vi "Measurement Logic.vi"() -> ()   [LabVIEW 2021, in "audio_acMeasurement.lvlib"]
uses:
  audio_acMeasurement.lvlib
  Measurement Configuration.ctl
  <vilib>/MeasurementLink/MeasurementLink Measurement Server/Classes/MeasurementContext/MeasurementContext.lvclass
  Measurement Results.ctl
  <vilib>/PDM Acquisition Toolkit/host/Classes/Tasks/PCM Input/Controls/DVR PCM Input Task.ctl
  <vilib>/PDM Acquisition Toolkit/host/Classes/Tasks/PCM Input/PCM Input Task.lvclass
  <vilib>/DAQmx/create/channels.llb/DAQmx Create Channel (AO-Voltage-Basic).vi
  <vilib>/DAQmx/configure/timing.llb/DAQmx Timing (Sample Clock).vi
  <vilib>/DAQmx/create/channels.llb/DAQmx Create Channel (AO-FuncGen).vi
  <vilib>/PDM Acquisition Toolkit/host/API/Public/Start/Start PCM Input Task.vi
  <vilib>/PDM Acquisition Toolkit/host/API/Public/Read/Read PCM Input Waveform.vi
  <vilib>/PDM Acquisition Toolkit/host/API/Public/Clear/Clear PCM Input Task.vi
  <resource>/objmgr/daqmx.rc
  <vilib>/PDM Acquisition Toolkit/host/API/PDM Acquisition Toolkit.lvlib
panel:
  out "Measurement Results":T1
  out "Measurement Context out":refnum<class "MeasurementContext.lvclass">
  in  "Measurement Context":refnum<class "MeasurementContext.lvclass">
  in  "Measurement Configuration":T2={"Band start"=20.0, "Band stop"=20000.0, "Weighting filter"=0, "Full scale range"=3.16, "Analog source resource name"="", "Frequency"=1000.0, "Amplitude"=1.0, "Protocol capture resource name"="PXI1Slot7\\I2Si 0", "Protocol capture channel"="", "Clock rate"=12288000, "Number of words"=19200, "Sensitivity"=0.34762, "JSONFile"=""}
  out "error out":errorcluster
  in  "error in":errorcluster
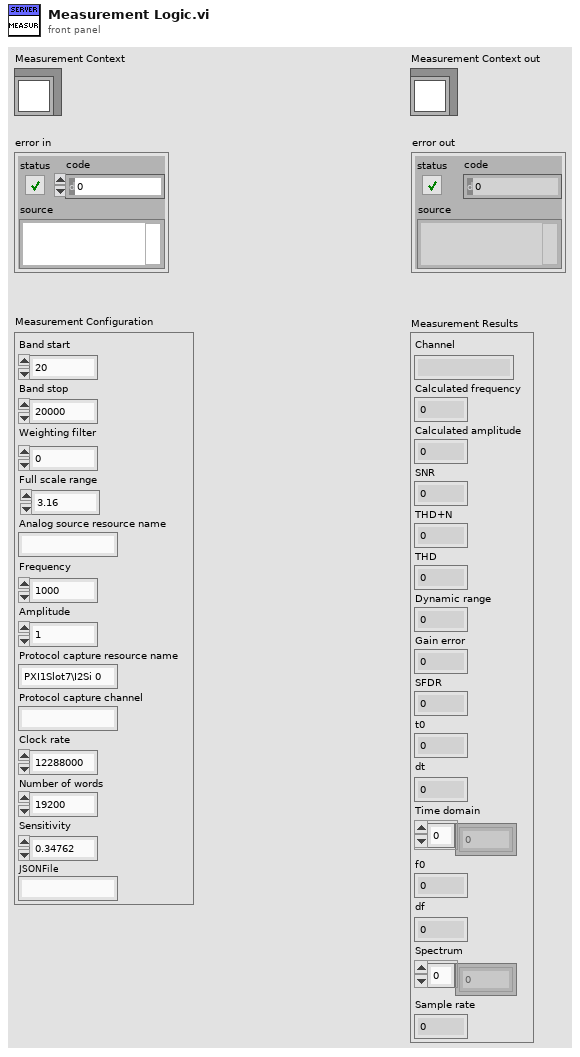
[diagram p1: front panel]
types:
  T1 = typedef "audio_acMeasurement.lvlib/Measurement Results.ctl" = cluster{"Channel":string, "Calculated frequency":dbl, "Calculated amplitude":dbl, "SNR":dbl, "THD+N":dbl, "THD":dbl, "Dynamic range":dbl, "Gain error":dbl, "SFDR":dbl, "t0":dbl, "dt":dbl, "Time domain":dbl[], "f0":dbl, "df":dbl, "Spectrum":dbl[], "Sample rate":u32}
  T2 = typedef "audio_acMeasurement.lvlib/Measurement Configuration.ctl" = cluster{"Band start":dbl, "Band stop":dbl, "Weighting filter":u16, "Full scale range":dbl, "Analog source resource name":string, "Frequency":dbl, "Amplitude":dbl, "Protocol capture resource name":string, "Protocol capture channel":string, "Clock rate":u32, "Number of words":u32, "Sensitivity":dbl, "JSONFile":string}
  T3 = typedef "PDM Acquisition Class Library.lvlib/PCM Input Task.lvclass/DVR PCM Input Task.ctl" = refnum<data-value>
  T4 = cluster{"DSG Session":refnum<k21>, "Calculated sample rate":u32, "PCM input task out":T3}
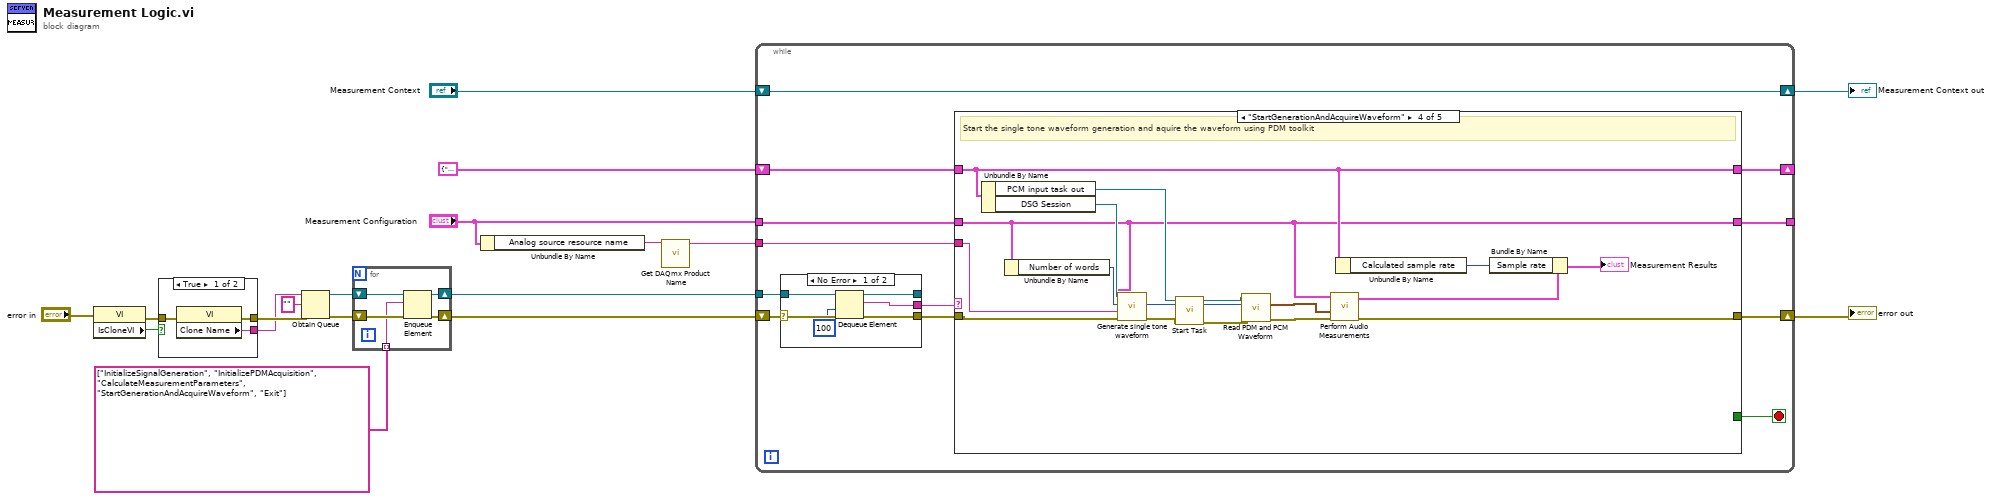
[diagram p0: block diagram]
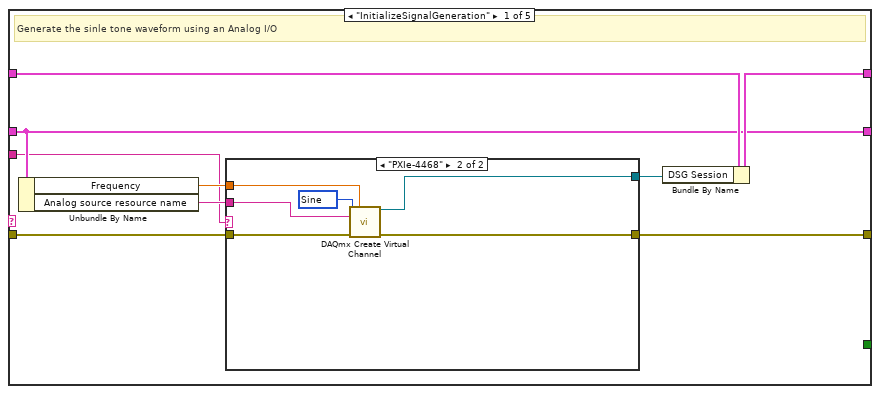
[diagram p2: hidden frame]
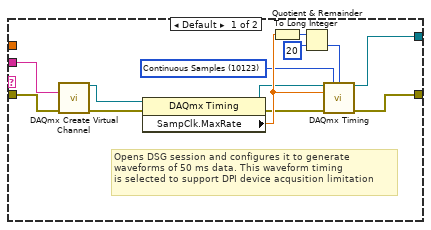
[diagram p3: hidden frame]
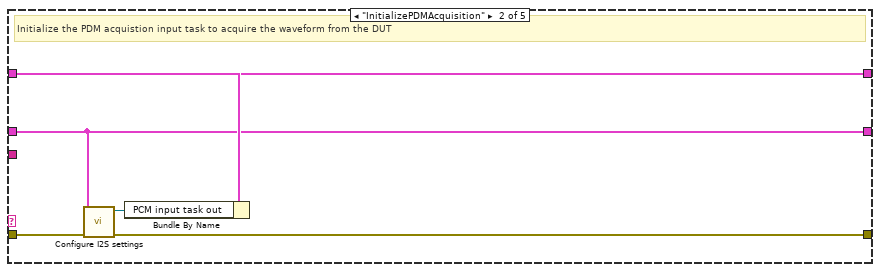
[diagram p4: hidden frame]
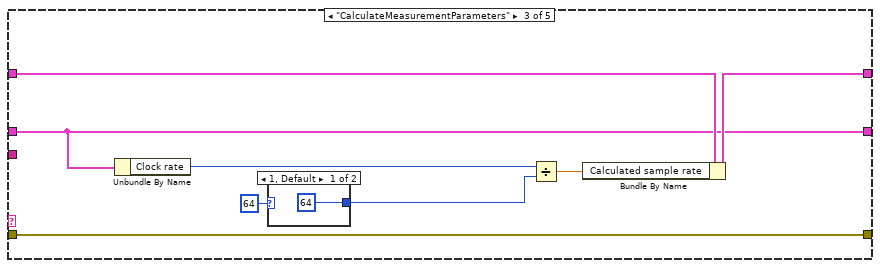
[diagram p5: hidden frame]
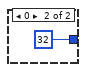
[diagram p6: hidden frame]
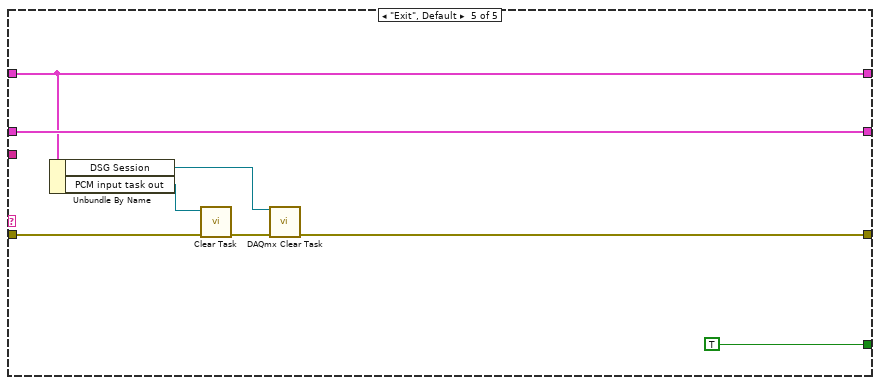
[diagram p7: hidden frame]
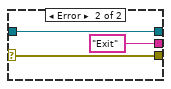
[diagram p8: hidden frame]
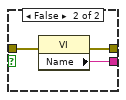
[diagram p9: hidden frame]
diagram:
  n1 = property class="VI"(error in="error in") -> (error out=w14:errorcluster, "IsCloneVI"=w15:bool)  [unwired: 1 in, 1 out]
  n2 = case shown="True" w15 {
    tunnel: [w21 w24] -> w13
    tunnel: [w20 w23] -> w12
    tunnel: w14 -> [w19 w22]
    frame True {
      n3 = property class="VI"(error in=w19) -> (error out=w21:errorcluster, "Clone Name"=w20:string)  [unwired: 1 in, 1 out]
    }
    frame False {
      n4 = property class="VI"(error in=w22) -> (error out=w24:errorcluster, "Name"=w23:string)  [unwired: 1 in, 1 out]
    }
  }
  n5 = Obtain Queue(name (unnamed)=w12, element data type="", error in (no error)=w13) -> (queue out=w17:refnum<queue>, error out=w11:errorcluster)  [unwired: 2 in, 1 out]
  n6 = for {
    shift-right: [w27] -> w10
    shift-left: w17 -> [w29]
    shift-right: [w26] -> w9
    shift-left: w11 -> [w28]
    tunnel: string[] ["InitializeSignalGeneration", "InitializePDMAcquisition", "CalculateMeasurementParameters", "StartGenerationAndAcquireWaveform", "Exit"] ("Step sequence") -> [w25] mode=indexing
    n7 = Enqueue Element(queue=w29, element=w25, error in (no error)=w28) -> (queue out=w27:refnum<queue>, error out=w26:errorcluster)  [unwired: 1 in, 1 out]
  }
  n8 = Unbundle By Name("Measurement Configuration") -> ("Analog source resource name"=w3:string)
  n9 = call "Get DAQmx Product Name.vi"("DAQmx resource name"=w3) -> ("DAQmx product type"=w1:string)  [unwired: 10 in]
  n10 = while {
    tunnel: w10 -> [w41]
    shift-right: [w38] -> w6
    shift-left: w9 -> [w37]
    shift-right: [w33] -> w4
    shift-left: "Measurement Context" -> [w33]
    tunnel: "Measurement Configuration" -> [w34]
    tunnel: [w35] -> _
    shift-right: [w31] -> _
    shift-left: T4 {"DSG Session"="", "Calculated sample rate"=0, "PCM input task out"=refnum} -> [w36]
    tunnel: w1 -> [w30]
    stop <- w32 stop-if-true
    n11 = case shown="No Error" w37 {
      selector: w37 -> [w113 w117]
      tunnel: w41 -> [w115 w116]
      tunnel: [w114 "Exit" ("t")] -> w40
      tunnel: [w112 w117] -> w39
      tunnel: [w110 w116] -> _
      frame No Error {
        n12 = Dequeue Element(queue=w115, timeout in ms (-1)=100, error in (no error)=w113) -> (queue out=w110:refnum<queue>, element=w114:string, error out=w112:errorcluster)  [unwired: 1 out]
      }
      frame Error {
      }
    }
    n13 = case shown="\"StartGenerationAndAcquireWaveform\"" w40 {
      tunnel: w39 -> [w49 w75 w78 w101 w108]
      tunnel: [w48 w72 w78 w98 w106] -> w38
      tunnel: w34 -> [w44 w70 w81 w88 w109]
      tunnel: w36 -> [w47 w74 w83 w94 w105]
      tunnel: [w45 w71 w82 w94 w105] -> w31
      tunnel: [w44 w70 w81 w88 w109] -> w35
      tunnel: [_ _ _ _ TRUE] -> w32
      tunnel: w30 -> [w42 _ _ w99 _]
      frame "InitializeSignalGeneration" {
        # "Generate the sinle tone waveform using an Analog I/O"
        n14 = Unbundle By Name(w44) -> ("Frequency"=w43:dbl, "Analog source resource name"=w50:string)
        n15 = case shown="\"PXIe-4468\"" w42 {
          tunnel: w50 -> [w63 w66]
          tunnel: w49 -> [w62 w69]
          tunnel: [w61 w68] -> w48
          tunnel: [w51 w67] -> w46
          tunnel: w43 -> [_ w64]
          frame Default {
            w52 = 10123 items=["Finite Samples"=10178, "Continuous Samples"=10123, "Hardware Timed Single Point"=12522] ("sample mode")
            # "Opens DSG session and configures it to generate\nwaveforms of 50 ms data. This waveform timing\nis selected to support DPI device acqusition limitation"
            n16 = call-poly <vilib>:"DAQmx Create Virtual Channel.vi"("physical channels"=w63, "error in"=w62) -> ("task out"=w60:refnum<k21>, "error out"=w59:errorcluster)  [unwired: 12 in]
            n17 = property class="DAQmx Timing"(reference=w60, error in=w59) -> (reference out=w55:refnum<k21>, error out=w56:errorcluster, "SampClk.MaxRate"=w57:dbl)
            n18 = To Long Integer(number=w57) -> (32bit integer=w53:i32)
            n19 = Quotient & Remainder(x=w53, y=20) -> (floor(x/y)=w58:i32)  [unwired: 1 out]
            n20 = call-poly <vilib>:"DAQmx Timing.vi"("task/channels in"=w55, "sample mode"=w52, "samples per channel"=w58, "rate"=w57, "error in"=w56) -> ("task out"=w51:refnum<k21>, "error out"=w61:errorcluster)  [unwired: 9 in]
          }
          frame "PXIe-4468" {
            w65 = 14751 items=["Sine"=14751, "Triangle"=14752, "Square"=14753, "Sawtooth"=14754] ("type")
            n21 = call-poly <vilib>:"DAQmx Create Virtual Channel.vi"("frequency"=w64, "physical channels"=w66, "type"=w65, "error in"=w69) -> ("task out"=w67:refnum<k21>, "error out"=w68:errorcluster)  [unwired: 10 in]
          }
        }
        n22 = Bundle By Name(cluster=w47, "DSG Session"=w46) -> (w45:T4)
      }
      frame "InitializePDMAcquisition" {
        # "Initialize the PDM acquistion input task to acquire the waveform from the DUT"
        n23 = call "Configure I2S settings.vi"("error in (no error)"=w75, "Measurement Configuration"=w70) -> ("error out"=w72:errorcluster, "PCM input task out"=w73:T3)  [unwired: 8 in]
        n24 = Bundle By Name(cluster=w74, "PCM input task out"=w73) -> (w71:T4)
      }
      frame "CalculateMeasurementParameters" {
        n25 = Unbundle By Name(w81) -> ("Clock rate"=w80:u32)
        n26 = case shown="1, Default" u16 64 ("Frame size") {
          tunnel: [64 32] -> w77
          frame 1, Default {
          }
          frame 0 {
          }
        }
        n27 = Divide(x=w80, y=w77) -> (x/y=w79:dbl)
        n28 = Bundle By Name(cluster=w83, "Calculated sample rate"=w79) -> (w82:T4)
      }
      frame "StartGenerationAndAcquireWaveform" {
        # "Start the single tone waveform generation and aquire the waveform using PDM toolkit"
        n29 = Unbundle By Name(w94) -> ("PCM input task out"=w93:T3, "DSG Session"=w100:refnum<k21>)
        n30 = Unbundle By Name(w88) -> ("Number of words"=w89:u32)
        n31 = call "Generate single tone waveform.vi"("error in (no error)"=w101, "DAQmx product type"=w99, "Measurement Configuration"=w88, "DSG task in"=w100) -> ("error out"=w87:errorcluster)  [unwired: 6 in, 1 out]
        n32 = call-poly <vilib>:"Start Task.vi"("error in"=w87, "PCM input task in"=w93) -> ("error out"=w90:errorcluster, "PCM input task out"=w92:T3)  [unwired: 8 in]
        n33 = call-poly <vilib>:"Read PDM and PCM Waveform.vi"("error in"=w90, "words per channel"=w89, "PCM input task In"=w92) -> ("error out"=w91:errorcluster, "PCM waveforms"=w86:waveform(dbl)[])  [unwired: 5 in, 2 out]
        n34 = call "Perform Audio Measurements.vi"("Measurement Configuration"=w88, "PCM waveforms"=w86, "error in (no error)"=w91) -> ("Measurement Results"=w97:T1, "error out"=w98:errorcluster)  [unwired: 6 in]
        n35 = Unbundle By Name(w94) -> ("Calculated sample rate"=w96:u32)
        n36 = Bundle By Name(cluster=w97, "Sample rate"=w96) -> (→"Measurement Results":T1)
      }
      frame "Exit", Default {
        n37 = Unbundle By Name(w105) -> ("DSG Session"=w104:refnum<k21>, "PCM input task out"=w103:T3)
        n38 = call-poly <vilib>:"Clear Task.vi"("error in"=w108, "PCM input task in"=w103) -> ("error out"=w107:errorcluster)  [unwired: 9 in]
        n39 = call <vilib>:"DAQmx Clear Task.vi"("task in"=w104, "error in"=w107) -> ("error out"=w106:errorcluster)  [unwired: 13 in]
      }
    }
  }
  "error out" <- w6
  "Measurement Context out" <- w4
